vi "WireToConnectorPane__slk_mt.vi"(5 "terminal index":u32, 6 "icon visible? (T)":bool=TRUE, 7 "pattern (no change: 0)":u32, 8 "error in (no error)":errorcluster, 10 "control refnum in":refnum<vi>, 11 "vi refnum in":refnum<vi>) -> (0 "error out":errorcluster, 3 "duplicated vi refnum out":refnum<vi>)   [LabVIEW 2015, in "Lazyboots Menu Tool.lvlib"]
doc: "Wires control to the specified terminal of connector pane."
uses:
  <vilib>/SLK/Lazyboots Menu Tool/Library/Lazyboots Menu Tool.lvlib
panel:
  # "WireToConnectorPane__slk_mt.vi\nWires control to the specified terminal of connector pane.\n\nNOTICE -- YOU MUST LEAVE THIS NOTICE IN PLACE.\n\nCopyright (c) 2011, LIANG LIU Shawn.Liu.cn@gmail.com\nAll rights reserved.\n\nRedistribution and use in source and binary forms, with or without modification, are permitted provided that the following conditions are met:\n-Redistributions of source code must retain the above copyright notice, this list of conditions and the following disclaimer.\n-Redistributions in binary form must reproduce the above copyright notice, this list of conditions and the following disclaimer in the documentation and/or other materials provided with the distribution.\n-Neither the name of the eLp nor the names of its contributors may be used to endorse or promote products derived from this software without specific prior written permission.\n\nTHIS SOFTWARE IS PROVIDED BY THE COPYRIGHT HOLDERS AND CONTRIBUTORS \"AS IS\" AND ANY EXPRESS OR IMPLIED WARRANTIES, INCLUDING, BUT NOT LIMITED TO, THE IMPLIED WARRANTIES OF MERCHANTABILITY AND FITNESS FOR A PARTICULAR PURPOSE ARE DISCLAIMED. IN NO EVENT SHALL THE COPYRIGHT HOLDER OR CONTRIBUTORS BE LIABLE FOR ANY DIRECT, INDIRECT, INCIDENTAL, SPECIAL, EXEMPLARY, OR CONSEQUENTIAL DAMAGES (INCLUDING, BUT NOT LIMITED TO, PROCUREMENT OF SUBSTITUTE GOODS OR SERVICES; LOSS OF USE, DATA, OR PROFITS; OR BUSINESS INTERRUPTION) HOWEVER CAUSED AND ON ANY THEORY OF LIABILITY, WHETHER IN CONTRACT, STRICT LIABILITY, OR TORT (INCLUDING NEGLIGENCE OR OTHERWISE) ARISING IN ANY WAY OUT OF THE USE OF THIS SOFTWARE, EVEN IF ADVISED OF THE POSSIBILITY OF SUCH DAMAGE."
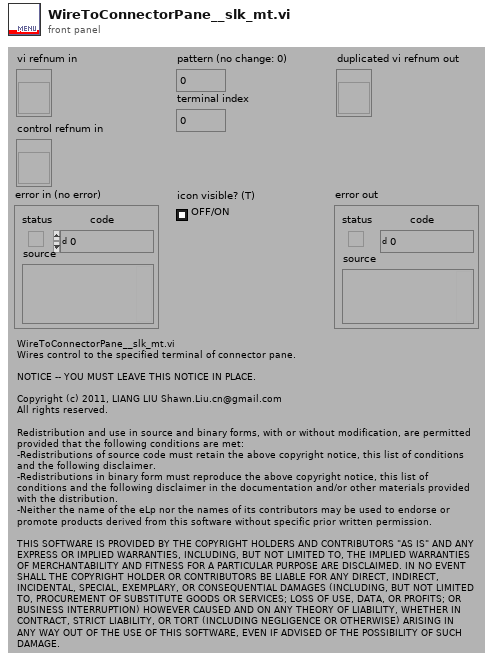
[diagram p1: front panel]
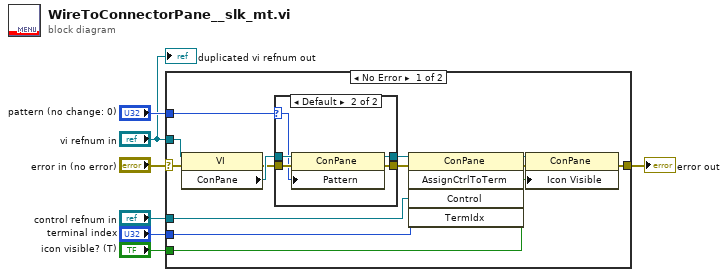
[diagram p0: block diagram]
diagram:
  n1 = case shown="No Error" "error in (no error)" {
    selector: "error in (no error)" -> [w16 w28]
    tunnel: "pattern (no change: 0)" -> [w15 _]
    tunnel: "vi refnum in" -> [w12 _]
    tunnel: "control refnum in" -> [w11 _]
    tunnel: "terminal index" -> [w10 _]
    tunnel: "icon visible? (T)" -> [w9 _]
    tunnel: [w8 w28] -> w2
    frame No Error {
      n2 = property class="VI"(reference=w12, error in=w16) -> (error out=w17:errorcluster, "ConPane"=w20:refnum<vi>)  [unwired: 1 out]
      n3 = case shown="Default" w15 {
        selector: w15 -> [_ w23]
        tunnel: w20 -> [w22 w27]
        tunnel: [w22 w26] -> w19
        tunnel: [w21 w25] -> w18
        tunnel: w17 -> [w21 w24]
        frame 0 {
        }
        frame Default {
          n4 = property class="ConPane"(reference=w27, error in=w24, "Pattern"=w23) -> (reference out=w26:refnum<vi>, error out=w25:errorcluster)
        }
      }
      n5 = invoke class="ConPane" method="AssignCtrlToTerm"(reference=w19, error in=w18, "Control"=w11, "TermIdx"=w10) -> (reference out=w13:refnum<vi>, error out=w14:errorcluster)  [unwired: 1 in, 3 out]
      n6 = property class="ConPane"(reference=w13, error in=w14, "Icon Visible"=w9) -> (error out=w8:errorcluster)  [unwired: 1 out]
    }
    frame Error {
    }
  }
  "error out" <- w2
  "duplicated vi refnum out" <- "vi refnum in"
